vi "testPixelFly2.vi"() -> ()   [LabVIEW 2009, in "run.lvlib"]
uses:
  testing/run.lvlib
  Tools/Filing/FileNeologist/FileNeologist.lvclass
panel:
  in  "number of images":i32=3
  out "Image":T1(plugin-control)
  in  "Save":bool=TRUE
  out "Board Parameters":T2 {"Vertical bin" items=["1", "2"]; "Horizontal bin" items=["1", "2"]}
  in  "gain":i32(ring) items=["Low (X1)", "High (X2)"]
  in  "exp time":i32(slide)=5 min=1 max=10000 scale=0.0..500.0
  in  "V bin":i32(ring) items=["1", "2"]
  in  "H bin":i32(ring) items=["1", "2"]
  in  "trigger":bool
  in  "Exposure mode":u16(ring)=2 items=["Asynch shutter", "Double shot", "Video mode", "Auto exposure"]
  out "ccdtemp":i32(slide) scale=0.0..100.0
  in  "stop":bool
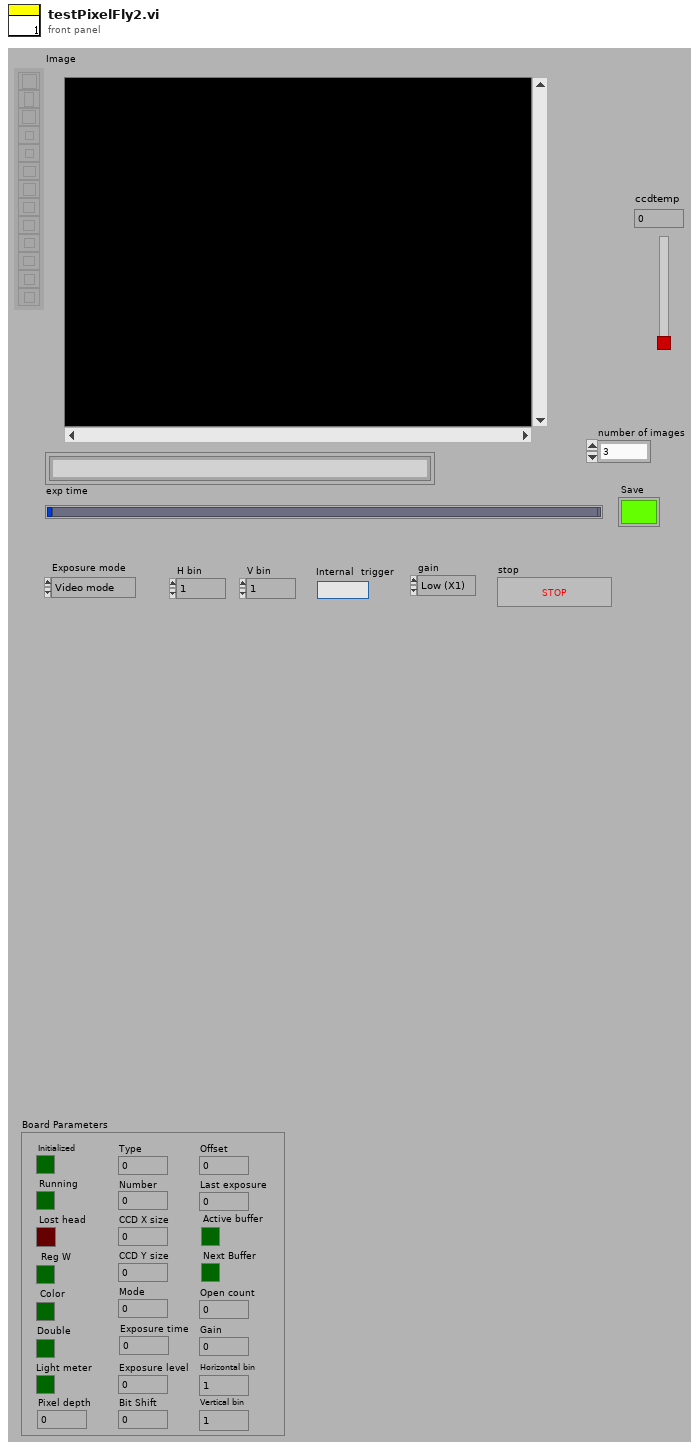
[diagram p1: front panel]
types:
  T1 = typedef "IMAQ Image.ctl" = refnum<image>
  T2 = cluster{"Type":u32, "Number":u32, "Initialized":bool, "Running":bool, "Lost head":bool, "CCD X size":u32, "CCD Y size":u32, "Mode":u32, "Exposure time":u32, "Exposure level":u32, "Horizontal bin":u32, "Vertical bin":u32, "Reg W":bool, "Gain":u32, "Pixel depth":i32, "Bit Shift":u32, "Offset":u32, "Last exposure":u32, "Double ":bool, "Light meter":bool, "Color":bool, "Open count":u32, "Active buffer":bool, "Next Buffer":bool}
  T3 = typedef "IMAQ Rectangle" = cluster{"Left":i32, "Top":i32, "Right":i32, "Bottom":i32, "Rotation":dbl}
  T4 = cluster{"Objects":u16, "Threshold":i32, "Reject Border":bool, "Fill Holes":bool, "Min Object Size":bool, "Min Size":i32, "Max Object Size":bool, "Max Size":i32, "Show Search Area":bool, "Show Center":bool, "Show Bounding Box":bool}
  T5 = cluster{"Left":i32, "Top":i32, "Right":i32, "Bottom":i32}
  T6 = typedef "Image Type" = u32
  T7 = cluster{"ccdxsize":i32, "ccdy":i32, "pictx":i32, "picty":i32, "bitspixel":i32}
  T8 = cluster{"Write":bool, "Write done":bool, "Queued":bool, "Cancelled":bool, "Select":bool, "Select done":bool, "Burst":bool, "Size":bool, "Event":bool, "Timeout":bool, "Open":i32, "Map":i32, "Exposure":i32[], "Offset":i32[], "Size":i32[], "Transfer":i32[], "Total Size":i32}
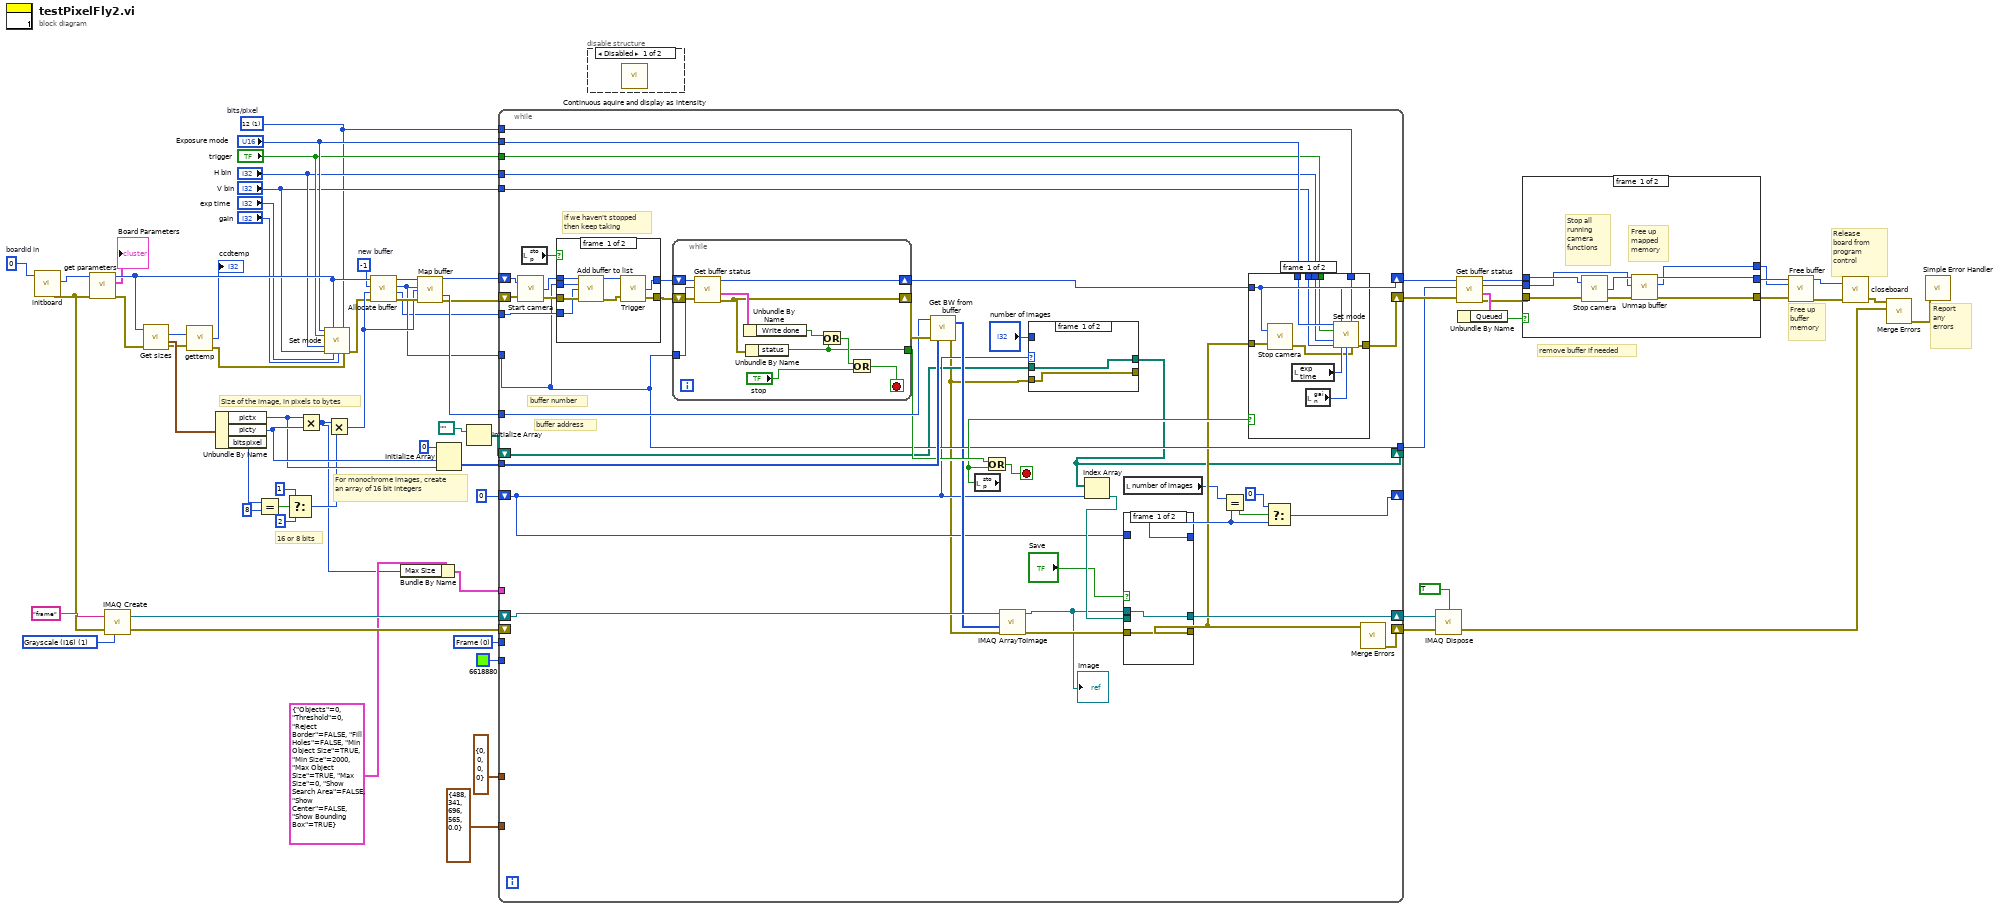
[diagram p0: block diagram]
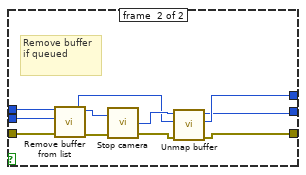
[diagram p3: hidden frame]
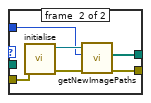
[diagram p4: hidden frame]
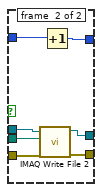
[diagram p5: hidden frame]
diagram:
  w9 = u32 0 items=["Frame", "Fill", "Highlight"] ("Drawing Mode (Frame)")
  w20 = T6 1 items=["Grayscale (U8)", "Grayscale (I16)", "Grayscale (SGL)", "Complex (CSG)", "RGB (U32)", "HSL (U32)", "RGB (U64)", "Grayscale (U16)"] ("Image Type")
  w32 = 1 items=["8", "12"]  # bits/pixel
  w48 = -1  # new buffer
  w53 = 0  # boardid in
  # "remove buffer if needed"
  # "Report any errors"
  # "Release board from program control"
  # "Free up buffer memory"
  # "16 or 8 bits"
  # "For monochrome images, create an array of 16 bit integers"
  # "Size of the image, in pixels to bytes"
  n1 = call <instrlib>:"initboard.vi"("boardid in"=w53) -> ("boardid"=w69:i32, "error out"=w21:errorcluster)  [unwired: 3 in, 1 out]
  n2 = call <instrlib>:"get parameters.vi"("error in (no error)"=w21, "Handle in"=w69) -> ("error out"=w57:errorcluster, "Board Parameters"=→"Board Parameters":T2, "Error out"=w54:i32)  [unwired: 2 in, 1 out]
  n3 = call "IMAQ Create"("Image Name"="frame", "Image Type"=w20, "error in (no error)"=w21) -> ("New Image"=w19:T1, "error out"=w18:errorcluster)  [unwired: 2 in]
  n4 = call <instrlib>:"Get sizes.vi"("Handle in"=w54, "error in (no error)"=w57) -> ("Handle out"=w55:i32, "Picture parameters"=w65:T7, "error out"=w56:errorcluster)  [unwired: 1 in, 1 out]
  n5 = call <instrlib>:"gettemp.vi"("Handle in"=w55, "error in (no error)"=w56) -> ("ccdtemp"=→"ccdtemp":i32, "error out"=w70:errorcluster)  [unwired: 1 out]
  n6 = Unbundle By Name(w65) -> ("pictx"=w62:i32, "picty"=w63:i32, "bitspixel"=w64:i32)
  n7 = Equal?(x=w64, y=8) -> (x = y?=w61:bool)
  n8 = Select(t=1, s=w61, f=2) -> (s? t:f=w58:i32)
  n9 = Multiply(x=w62, y=w63) -> (x*y=w4:i32)
  n10 = call <instrlib>:"Set mode.vi"("Exposure mode"="Exposure mode", "Handle in"=w54, "bits/pixel"=w32, "trigger"="trigger", "H bin"="H bin", "V bin"="V bin", "exp time"="exp time", "gain"="gain", "error in (no error)"=w70) -> ("error out"=w50:errorcluster)  [unwired: 6 in]
  n11 = Multiply(x=w4, y=w58) -> (x*y=w51:i32)
  n12 = call <instrlib>:"Allocate buffer.vi"("error in (no error)"=w50, "Size request"=w51, "Buffer request"=w48, "Handle in"=w54) -> ("error out"=w68:errorcluster, "Size"=w30:i32, "Buffer number"=w31:i32, "Handle out"=w71:i32)
  n13 = Bundle By Name(cluster=T4 {"Objects"=0, "Threshold"=0, "Reject Border"=FALSE, "Fill Holes"=FALSE, "Min Object Size"=TRUE, "Min Size"=2000, "Max Object Size"=TRUE, "Max Size"=0, "Show Search Area"=FALSE, "Show Center"=FALSE, "Show Bounding Box"=TRUE} ("Settings"), "Max Size"=w4) -> (w6:T4)
  n14 = call <instrlib>:"Map buffer.vi"("Handle in"=w71, "Buffer in"=w31, "size"=w51, "error in (no error)"=w68) -> ("Handle out"=w29:i32, "Buffer address"=w52:i32, "error out"=w28:errorcluster)  [unwired: 8 in, 1 out]
  n15 = Initialize Array(u16 0 ("16 bit integers"), w63, w62) -> (w49:u16[][])
  n16 = Initialize Array(path "") -> (w2:path[])  [unwired: 1 in]
  n17 = while {
    tunnel: w31 -> [w92]
    shift-right: [w97] -> w43
    shift-left: w29 -> [w96]
    shift-right: [w98] -> w42
    shift-left: w28 -> [w90]
    tunnel: w52 -> [w108]
    tunnel: w49 -> [w107]
    tunnel: "Exposure mode" -> [w102]
    tunnel: "trigger" -> [w101]
    tunnel: "H bin" -> [w100]
    tunnel: "V bin" -> [w99]
    tunnel: w32 -> [w103]
    tunnel: w30 -> [w106]
    tunnel: [w92] -> w26
    shift-right: [w88] -> w17
    shift-left: w19 -> [w91]
    shift-right: [w89] -> w16
    shift-left: w18 -> [_]
    tunnel: T5 {"Left"=0, "Top"=0, "Right"=0, "Bottom"=0} ("Rectangle") -> [_]
    tunnel: u32 6618880 -> [_]
    tunnel: w9 -> [_]
    tunnel: w6 -> [_]
    tunnel: T3 {"Left"=488, "Top"=341, "Right"=696, "Bottom"=565, "Rotation"=0.0} ("Rectangle") -> [_]
    shift-right: [w86] -> _
    shift-left: 0 -> [w77]
    shift-right: [w75] -> _
    shift-left: w2 -> [w76]
    stop <- w104 stop-if-true
    # "buffer address"
    # "buffer number"
    # "if we haven't stopped\nthen keep taking"
    n18 = call <instrlib>:"Start camera.vi"("Handle in"=w96, "error in (no error)"=w90) -> ("Handle out"=w95:i32, "error out"=w94:errorcluster)  [unwired: 1 out]
    n19 = local read "stop"() -> (w112:bool)
    n20 = case shown="False" w112 {
      tunnel: w94 -> [w149 w150]
      tunnel: [w147 w150] -> w111
      tunnel: w95 -> [w146 w151]
      tunnel: [w144 w151] -> w110
      tunnel: w92 -> [w143 _]
      tunnel: w106 -> [w142 _]
      frame #0 {
        n21 = call <instrlib>:"Add buffer to list.vi"("Handle in"=w146, "Buffer in"=w143, "size"=w142, "error in (no error)"=w149) -> ("Handle out"=w145:i32, "error out"=w148:errorcluster)  [unwired: 9 in, 1 out]
        n22 = call <instrlib>:"Trigger.vi"("Handle in"=w145, "error in (no error)"=w148) -> ("Handle out"=w144:i32, "error out"=w147:errorcluster)  [unwired: 1 out]
      }
      frame #1 {
      }
    }
    n23 = while {
      tunnel: w92 -> [w155]
      shift-right: [w153] -> w97
      shift-left: w110 -> [w156]
      shift-right: [w154] -> w109
      shift-left: w111 -> [w157]
      tunnel: [w152] -> w105
      stop <- w158 stop-if-true
      n24 = call <instrlib>:"Get buffer status.vi"("error in (no error)"=w157, "Buffer request"=w155, "Handle in"=w156) -> ("error out"=w154:errorcluster, "Buffer status"=w162:T8, "Handle out"=w153:i32)  [unwired: 1 in, 1 out]
      n25 = Unbundle By Name(w162) -> ("Write done"=w161:bool)
      n26 = Unbundle By Name(w154) -> ("status"=w152:bool)
      n27 = Or(x=w161, y=w152) -> (x .or. y?=w160:bool)
      n28 = Or(x=w160, y="stop") -> (x .or. y?=w158:bool)
    }
    n29 = call <instrlib>:"Get BW from buffer.vi"("error in (no error)"=w109, "Array input"=w107, "Buffer address"=w108) -> ("error out"=w74:errorcluster, "Image data"=w78:u16[][])
    n30 = local read "stop"() -> (w93:bool)
    n31 = Or(x=w105, y=w93) -> (x .or. y?=w104:bool)
    n32 = call "IMAQ ArrayToImage"("error in (no error)"=w74, "Image Pixels (I16)"=w78, "Image"=w91) -> ("error out"=w82:errorcluster, "Image Out"=w79:T1)  [unwired: 7 in]
    "Image" <- w79
    n33 = case shown="0" w77 {
      tunnel: [w114 w118] -> w75
      tunnel: w76 -> [w114 _]
      tunnel: w74 -> [w113 w117]
      tunnel: [w113 w116] -> _
      tunnel: "number of images" -> [_ w115]
      frame #0 {
      }
      frame #1 {
        n34 = call "initialise.vi"("error in (no error)"=w117) -> ("error out"=w119:errorcluster, "FileNeologist out"=w120:refnum<class "FileNeologist.lvclass">)  [unwired: 9 in]
        n35 = call "getNewImagePaths.vi"("error in (no error)"=w119, "numberOfImages"=w115, "FileNeologist in"=w120) -> ("error out"=w116:errorcluster, "Paths"=w118:path[])  [unwired: 6 in, 1 out]
      }
    }
    n36 = Index Array(array=w75, index=w77) -> (element=w87:path)
    n37 = local read "number of images"() -> (w72:i32)
    n38 = case shown="True" "Save" {
      tunnel: [w122 w129] -> w88
      tunnel: [w121 w128] -> w81
      tunnel: w87 -> [_ w127]
      tunnel: w77 -> [_ w126]
      tunnel: [_ w125] -> w84
      tunnel: w82 -> [w121 w124]
      tunnel: w79 -> [w122 w123]
      frame #0 {
      }
      frame #1 {
        n39 = call-poly "IMAQ Write File 2"("error in (no error)"=w124, "File Path"=w127, "Image"=w123) -> ("error out"=w128:errorcluster, "Image Out (duplicate)"=w129:T1)  [unwired: 7 in]
        n40 = Increment(x=w126) -> (x+1=w125:i32)
      }
    }
    n41 = Equal?(x=w72, y=w84) -> (x = y?=w85:bool)
    n42 = case shown="False" w93 {
      tunnel: w103 -> [w140 _]
      tunnel: w102 -> [w139 _]
      tunnel: w101 -> [w138 _]
      tunnel: w100 -> [w137 _]
      tunnel: w99 -> [w136 _]
      tunnel: [w133 w141] -> w98
      tunnel: w81 -> [w132 w141]
      tunnel: w97 -> [w130 _]
      frame #0 {
        n43 = call <instrlib>:"Stop camera.vi"("Handle in"=w130, "error in (no error)"=w132) -> ("error out"=w131:errorcluster)  [unwired: 2 out]
        n44 = local read "exp time"() -> (w135:i32)
        n45 = local read "gain"() -> (w134:i32)
        n46 = call <instrlib>:"Set mode.vi"("Exposure mode"=w139, "Handle in"=w130, "bits/pixel"=w140, "trigger"=w138, "H bin"=w137, "V bin"=w136, "exp time"=w135, "gain"=w134, "error in (no error)"=w131) -> ("error out"=w133:errorcluster)  [unwired: 6 in]
      }
      frame #1 {
      }
    }
    n47 = Select(t=0, s=w85, f=w84) -> (s? t:f=w86:i32)
    n48 = call <vilib>:"Merge Errors.vi"("error in 1 (no error)"=w81) -> ("error out"=w89:errorcluster)  [unwired: 6 in]
  }
  n49 = disable-structure shown="Disabled" {
    frame #0 {
      n50 = call <instrlib>:"Continuous aquire and display as intensity.vi"() -> ()  [unwired: 1 in]
    }
    frame #1 {
    }
  }
  n51 = call "IMAQ Dispose"("All Images? (No)"=TRUE, "Image"=w17, "error in (no error)"=w16) -> ("error out"=w12:errorcluster)  [unwired: 3 in]
  n52 = call <instrlib>:"Get buffer status.vi"("error in (no error)"=w42, "Buffer request"=w26, "Handle in"=w43) -> ("error out"=w44:errorcluster, "Buffer status"=w45:T8, "Buffer number"=w41:i32, "Handle out"=w40:i32)  [unwired: 1 in]
  n53 = Unbundle By Name(w45) -> ("Queued"=w27:bool)
  n54 = case shown="True" w27 {
    tunnel: w44 -> [w167 w181]
    tunnel: [w165 w171] -> w23
    tunnel: w41 -> [w166 w180]
    tunnel: w40 -> [w168 w179]
    tunnel: [w164 w172] -> w25
    tunnel: [w163 w173] -> w24
    frame #0 {
      # "Free up mapped memory"
      # "Stop all running camera functions"
      n55 = call <instrlib>:"Stop camera.vi"("Handle in"=w168, "error in (no error)"=w167) -> ("Handle out"=w170:i32, "error out"=w169:errorcluster)  [unwired: 1 out]
      n56 = call <instrlib>:"Unmap buffer.vi"("error in (no error)"=w169, "Buffer in"=w166, "Handle in"=w170) -> ("error out"=w165:errorcluster, "Buffer number"=w163:i32, "Handle out"=w164:i32)  [unwired: 2 in]
    }
    frame #1 {
      # "Remove buffer if queued"
      n57 = call <instrlib>:"Remove buffer from list.vi"("error in (no error)"=w181, "Buffer in"=w180, "Handle in"=w179) -> ("error out"=w178:errorcluster, "Buffer number"=w174:i32, "Handle out"=w177:i32)  [unwired: 2 in]
      n58 = call <instrlib>:"Stop camera.vi"("Handle in"=w177, "error in (no error)"=w178) -> ("Handle out"=w175:i32, "error out"=w176:errorcluster)  [unwired: 1 out]
      n59 = call <instrlib>:"Unmap buffer.vi"("error in (no error)"=w176, "Buffer in"=w174, "Handle in"=w175) -> ("error out"=w171:errorcluster, "Buffer number"=w173:i32, "Handle out"=w172:i32)  [unwired: 2 in]
    }
  }
  n60 = call <instrlib>:"Free buffer.vi"("error in (no error)"=w23, "Buffer in"=w24, "Handle in"=w25) -> ("error out"=w46:errorcluster, "Handle out"=w39:i32)  [unwired: 2 in, 1 out]
  n61 = call <instrlib>:"closeboard.vi"("Handle in"=w39, "error in (no error)"=w46) -> ("error out"=w14:errorcluster)  [unwired: 2 out]
  n62 = call <vilib>:"Merge Errors.vi"("error in 2 (no error)"=w12, "error in 1 (no error)"=w14) -> ("error out"=w13:errorcluster)  [unwired: 5 in]
  n63 = call <vilib>:"Simple Error Handler.vi"("error in (no error)"=w13) -> ()  [unwired: 4 in, 5 out]
